vi "Inverter_JSON_step editor.vi"() -> ()   [LabVIEW 2020]
uses:
  controls/Inverter_step.ctl
  controls/Inverter_step_type.ctl
  MPB/controls/data type.ctl
  MPB/controls/write_read.ctl
panel:
  in  "read json file":bool
  in  "clear array":bool
  in  "save":bool
  out "steps array out":T1[](array[typedef]) {"dbl" format="%.3f"}
  in  "exit without saving":bool
  in  "steps array out":T1[](array[typedef]) {"dbl" format="%.3f"}
  in  "exit and save":bool
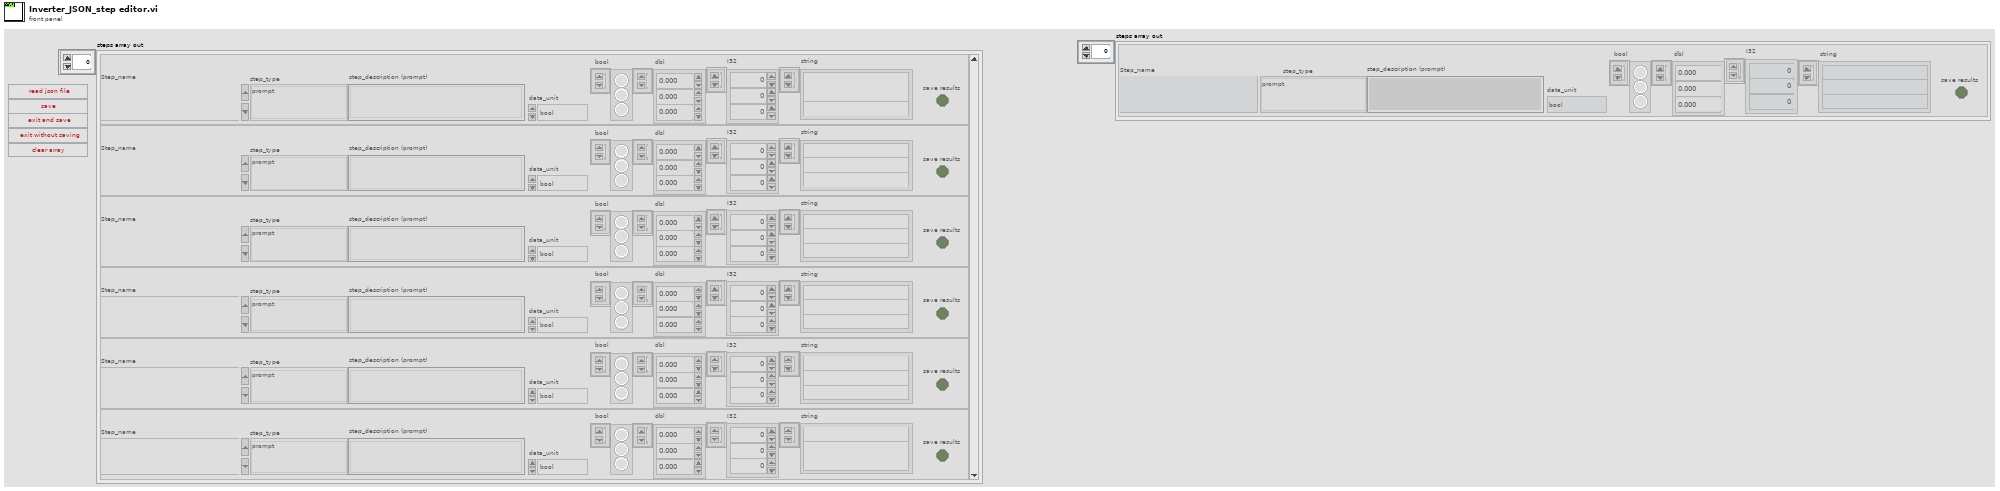
[diagram p1: front panel]
types:
  T1 = typedef "Inverter_step.ctl" = cluster{"step_description (prompt)":string, "save results":bool, "step_type":T2, "Step_name":string, "bool":bool[], "data_unit":T3, "dbl":dbl[], "I32":i32[], "string":string[]}
  T2 = typedef "Inverter_step_type.ctl" = enum16{"default", "prompt", "12V_power supply on_off", "write_PLC", "read_PLC", "wait (sec)", "record_pass_fail"}
  T3 = typedef "data type.ctl" = enum16{"bool", "string", "I32", "DBL"}
  T4 = typedef "write_read.ctl" = enum16{"write", "read"}
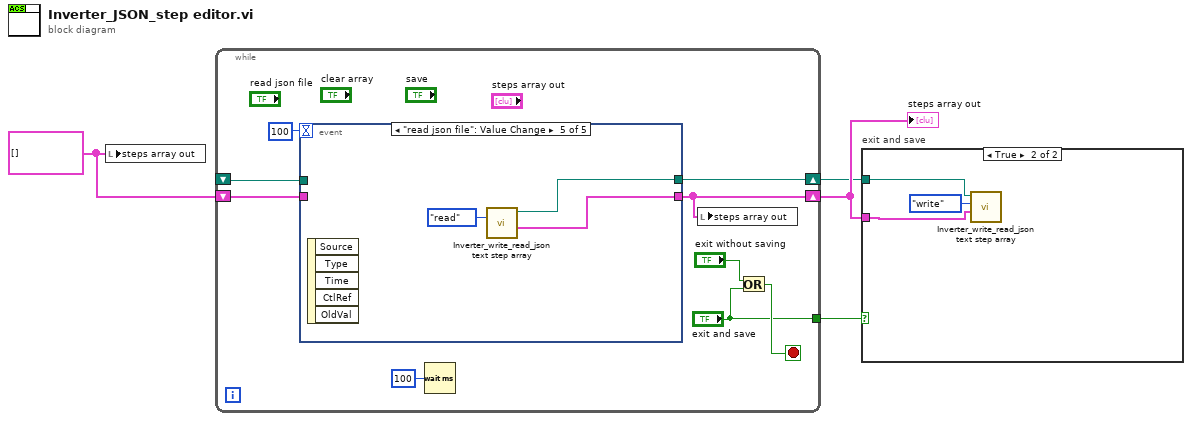
[diagram p0: block diagram]
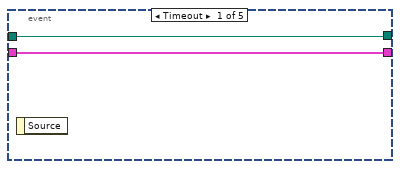
[diagram p3: hidden frame]
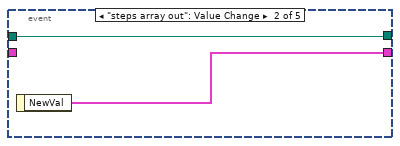
[diagram p4: hidden frame]
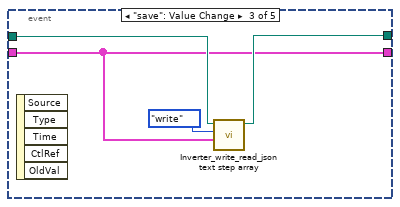
[diagram p5: hidden frame]
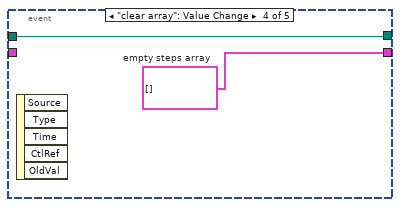
[diagram p6: hidden frame]
diagram:
  w1 = T1[] [] ("steps array out")
  n1 = local write "steps array out"(w1) -> ()
  n2 = while {
    shift-right: [w10] -> w3
    shift-left: w1 -> [w12]
    tunnel: ["exit and save"] -> w4
    shift-right: [w5] -> w2
    shift-left: _ -> [w6]
    stop <- w9 stop-if-true
    n3 = event shown="[4] \"read json file\": Value Change" {
      selector: _ -> [_ _ _ _ _]
      dyn-events: _ -> [_ _ _ _ _]
      timeout: 100 -> [_ _ _ _ _]
      tunnel: w12 -> [w15 _ w18 _ _]
      tunnel: [w15 w17 w18 w23 w24] -> w10
      tunnel: w6 -> [w14 w16 w19 w22 _]
      tunnel: [w14 w16 w20 w22 w25] -> w5
      event Timeout {
        n4 = event-data() -> ()  [unwired: 1 in, 1 out]
      }
      event "steps array out": Value Change {
        n5 = event-data() -> ("NewVal"=w17:T1[])  [unwired: 1 in]
      }
      event "save": Value Change {
        n6 = event-data() -> ()  [unwired: 1 in, 5 out]
        n7 = call "Inverter_write_read_json text step array.vi"("json_array_from_file"=w18, "write_read"=write_read."write", "File Path"=w19) -> ("File Path"=w20:path)  [unwired: 6 in, 2 out]
      }
      event "clear array": Value Change {
        w23 = T1[] []  # empty steps array
        n8 = event-data() -> ()  [unwired: 1 in, 5 out]
      }
      event "read json file": Value Change {
        n9 = event-data() -> ()  [unwired: 1 in, 5 out]
        n10 = call "Inverter_write_read_json text step array.vi"("write_read"=write_read."read") -> ("steps array out"=w24:T1[], "File Path"=w25:path)  [unwired: 8 in, 1 out]
      }
    }
    n11 = Wait (ms)(milliseconds to wait=u32 100) -> ()  [unwired: 1 out]
    n12 = local write "steps array out"(w10) -> ()
    n13 = Or(x="exit without saving", y="exit and save") -> (x .or. y?=w9:bool)
  }
  "steps array out" <- w3
  n14 = case "exit and save" shown="True" w4 {
    tunnel: w3 -> [_ w27]
    tunnel: w2 -> [_ w28]
    frame False {
    }
    frame True {
      n15 = call "Inverter_write_read_json text step array.vi"("json_array_from_file"=w27, "write_read"=write_read."write", "File Path"=w28) -> ()  [unwired: 6 in, 3 out]
    }
  }
